vi "Arm_XYZ_Constants.vi"() -> (1 "Unextended Length (in)":dbl, 3 "Pivot Height (in)":dbl)   [LabVIEW 2020]
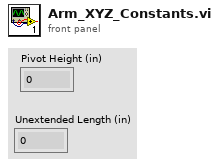
[diagram p1: front panel]
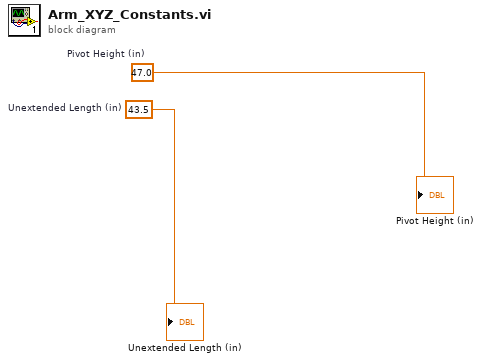
[diagram p0: block diagram]
diagram:
  w2 = 47.0  # Pivot Height (in)
  w1 = 43.5  # Unextended Length (in)
  "Pivot Height (in)" <- w2
  "Unextended Length (in)" <- w1
